vi "ArrayIterator_Create.vi"(8 "error in (no error)":errorcluster, 10 "BrowerComponents":refnum<class "BrowerComponent.lvclass">[](array[class]), 11 "reference in":refnum<class "ArrayIterator.lvclass">) -> (0 "error out":errorcluster, 3 "reference out":refnum<class "ArrayIterator.lvclass">)   [LabVIEW 2015, in "ArrayIterator.lvclass"]
uses:
  ArrayIterator.lvclass
  BrowerComponent/BrowerComponent/BrowerComponent.lvclass
  ArrayIterator.lvclass/ArrayIterator.ctl
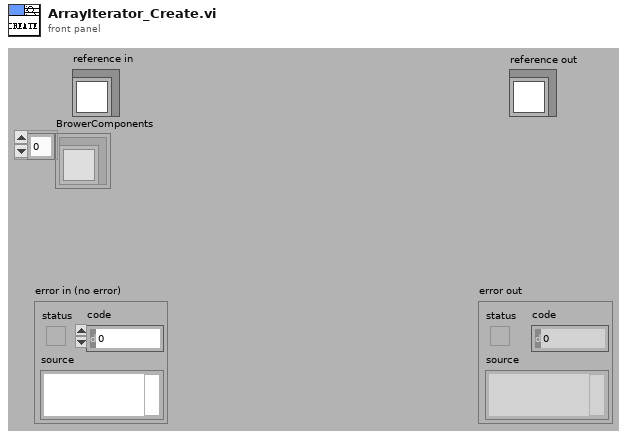
[diagram p1: front panel]
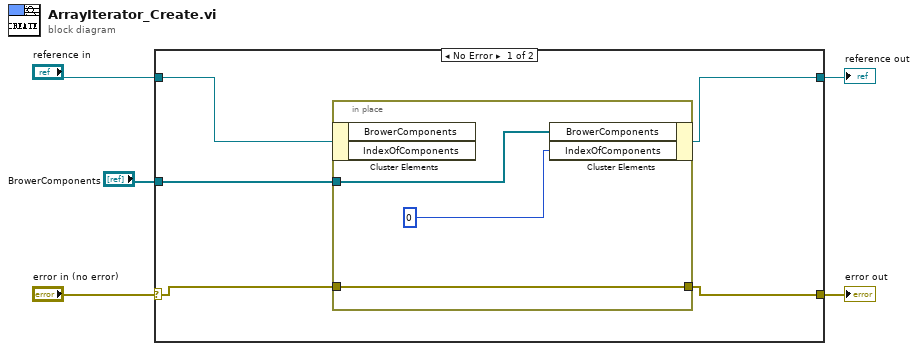
[diagram p0: block diagram]
diagram:
  n1 = case shown="No Error" "error in (no error)" {
    selector: "error in (no error)" -> [w10 w15]
    tunnel: [w9 w15] -> w4
    tunnel: "reference in" -> [w7 w14]
    tunnel: [w6 w14] -> w2
    tunnel: "BrowerComponents" -> [w8 _]
    frame No Error {
      n2 = in-place {
        in-place-border: w10 -> [w13]
        in-place-border: [w13] -> w9
        in-place-border: w8 -> [w12]
        n3 = in-place-cluster #1(w7) -> ()  [unwired: 2 out]
        n4 = in-place-cluster #1("BrowerComponents"=w12, "IndexOfComponents"=0) -> (w6:refnum<class "ArrayIterator.lvclass">)
      }
    }
    frame Error {
    }
  }
  "error out" <- w4
  "reference out" <- w2
